vi "SERIAL_BufferLoop.vi"(11 "navX DevRef":T1={"SerialPortRef"={"DevStatus"={"status"=FALSE, "code"=0, "source"=""}, "Serial Port Name"=""}, "Board Information"={"WhoAmI (50 | 0x32)"=0, "Board Revision"=0, "Firmware Major Version"=0, "Firmware Minor Version"=0}, "Status"={"Update Rate Hz"=0, "Accelerometer Full-Scale Range"=0, "Gyro Full-Scale Range"=0, "NAVX_OP_STATUS"=0, "NAVX_CAL_STATUS"=0, "NAVX_SELFTEST_STATUS"=0, "NAVX_SENSOR_STATUS"={"MOVING"=FALSE, "YAW_STABLE"=FALSE, "MAG_DISTURBANCE"=FALSE, "ALTITUDE_VALID"=FALSE, "SEALEVEL_PRESS_SET"=FALSE, "FUSED_HEADING_VALID"=FALSE}}, "Offsets"={"Yaw"=0.0, "Quat W"=0.0, "Quat X"=0.0, "Quat Y"=0.0, "Quat Z"=0.0}, "Update Rate (4Hz-60Hz)"=50, "Nav6Mode (YPR)"=enum."YPR", "refnum name"="", "error"={"status"=FALSE, "code"=0, "source"=""}, "Loop VI Refnum"=refnum} {"Status"."NAVX_OP_STATUS" items=["INITIALIZING", "SELFTEST_IN_PROGRESS", "ERROR", "IMU_AUTOCAL_IN_PROGRESS", "NORMAL"]; "Status"."NAVX_CAL_STATUS" items=["IMU_CAL_STATE_MASK"=3, "IMU_CAL_INPROGRESS"=0, "IMU_CAL_ACCUMULATE"=1, "IMU_CAL_COMPLETE"=2, "MAG_CAL_COMPLETE"=4, "BARO_CAL_COMPLETE"=8]}) -> ()   [LabVIEW 2014, in "navX-MXP IMU.lvlib"]
uses:
  navX-MXP IMU.lvlib
  Internal/navX Serial DevRef.ctl
  <vilib>/Rock Robotics/WPI/SerialPort/WPI_SerialPortRef.ctl
  COMMON/TypeDefs/Data TypeDefs/navX Board Information.ctl
  COMMON/TypeDefs/Data TypeDefs/navX Status Data.ctl
  COMMON/TypeDefs/Value TypeDefs/navX NAVX_OP_STATUS.ctl
  COMMON/TypeDefs/Value TypeDefs/navX NAVX_CAL_STATUS.ctl
  COMMON/TypeDefs/Value TypeDefs/navX NAVX_SENSOR_STATUS.ctl
  TypeDefs/navX Serial Mode.ctl
  <vilib>/Platform/TimedLoop/XDataNode/timing_clust.ctl
  <vilib>/Platform/TimedLoop/XDataNode/nitl_modes.ctl
  <vilib>/Platform/TimedLoop/XDataNode/wakeup.ctl
  <vilib>/platform/TimedLoop/XDataNode/XDataNode.xnode
  <vilib>/Platform/TimedLoop/XDataNode/XDNodeRunTimeDep.lvlib
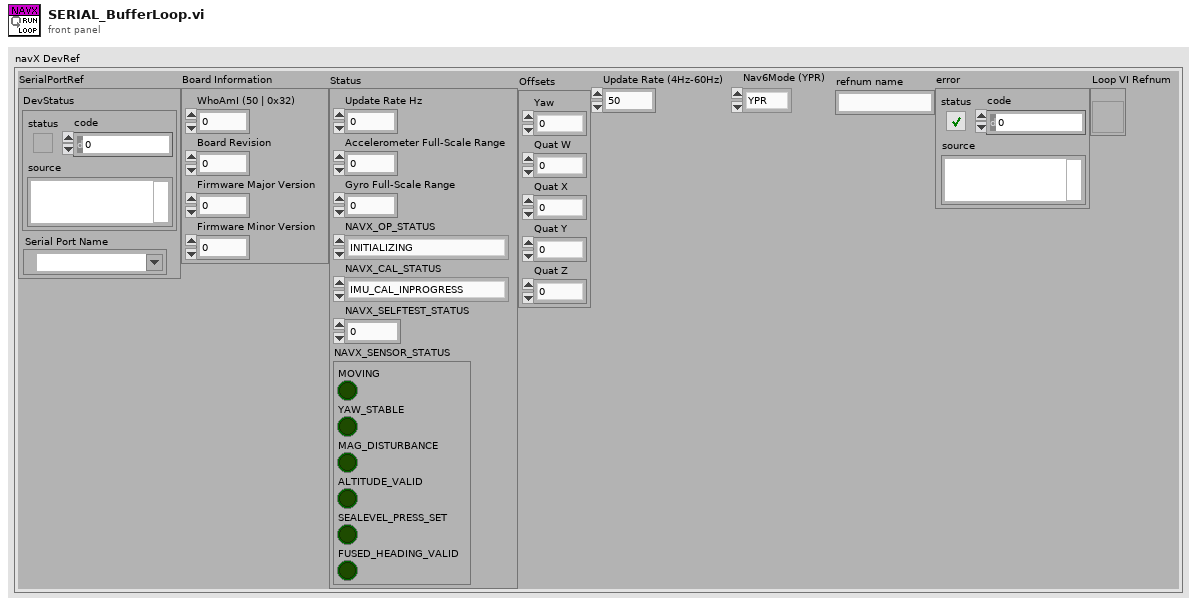
[diagram p1: front panel]
types:
  T1 = typedef "navX-MXP IMU.lvlib/navX Serial DevRef.ctl" = cluster{"SerialPortRef":T2, "Board Information":T3, "Status":T4, "Offsets":cluster{"Yaw":dbl, "Quat W":dbl, "Quat X":dbl, "Quat Y":dbl, "Quat Z":dbl}, "Update Rate (4Hz-60Hz)":u8, "Nav6Mode (YPR)":T8, "refnum name":string, "error":errorcluster, "Loop VI Refnum":refnum<vi>}
  T2 = typedef "WPI_SerialPortRef.ctl" = cluster{"DevStatus":errorcluster, "Serial Port Name":refnum<visa-resource-name>}
  T3 = typedef "navX-MXP IMU.lvlib/navX Board Information.ctl" = cluster{"WhoAmI (50 | 0x32)":u8, "Board Revision":u8, "Firmware Major Version":u8, "Firmware Minor Version":u8}
  T4 = typedef "navX-MXP IMU.lvlib/navX Status Data.ctl" = cluster{"Update Rate Hz":u8, "Accelerometer Full-Scale Range":u8, "Gyro Full-Scale Range":u16, "NAVX_OP_STATUS":T5, "NAVX_CAL_STATUS":T6, "NAVX_SELFTEST_STATUS":u8, "NAVX_SENSOR_STATUS":T7}
  T5 = typedef "navX-MXP IMU.lvlib/navX NAVX_OP_STATUS.ctl" = u8
  T6 = typedef "navX-MXP IMU.lvlib/navX NAVX_CAL_STATUS.ctl" = u8
  T7 = typedef "navX-MXP IMU.lvlib/navX NAVX_SENSOR_STATUS.ctl" = cluster{"MOVING":bool, "YAW_STABLE":bool, "MAG_DISTURBANCE":bool, "ALTITUDE_VALID":bool, "SEALEVEL_PRESS_SET":bool, "FUSED_HEADING_VALID":bool}
  T8 = typedef "navX-MXP IMU.lvlib/navX Serial Mode.ctl" = enum16{"YPR", "Gyro", "Quaternion"}
  T9 = typedef "XDNodeRunTimeDep.lvlib/timing_clust.ctl" = cluster{"Expected End [f-1]":u64, "Actual End [f-1]":u64, "Finished Late? [f-1]":bool, "Expected End [i-1]":u64, "Actual End [i-1]":u64, "Finished Late? [i-1]":bool, "Expected Start [i]":u64, "Actual Start [i]":u64, "Expected Start [f]":u64, "Actual Start [f]":u64, "Source Name":string, "Structure Name":string, "Period":i64, "Deadline":i64, "Offset":i64, "Start":i64, "Priority":i32, "Timeout":i32, "Mode":T10, "Wakeup Reason":T11, "Error":errorcluster, "Source Type":string, "Secondary Source Type":string, "Global End Time":u64, "Global Start Time":u64, "Frame Duration":u64, "Iteration Duration":u64, "Assigned CPU":i32, "I/O Scan Engine Mode":u32}
  T10 = typedef "XDNodeRunTimeDep.lvlib/nitl_modes.ctl" = enum32{"No Change", "Process missed periods, maintain original phase", "Discard missed periods, maintain original phase", "Process missed periods, ignore original phase", "Discard missed periods, ignore original phase"}
  T11 = typedef "XDNodeRunTimeDep.lvlib/wakeup.ctl" = enum32{"Normal", "Aborted", "Asynchronous wakeup", "Timing source error", "Timed loop error", "Timeout"}
  T12 = typedef "navX-MXP IMU.lvlib/navX YPRH Data.ctl" = cluster{"Yaw":dbl, "Pitch":dbl, "Roll":dbl, "Heading":dbl}
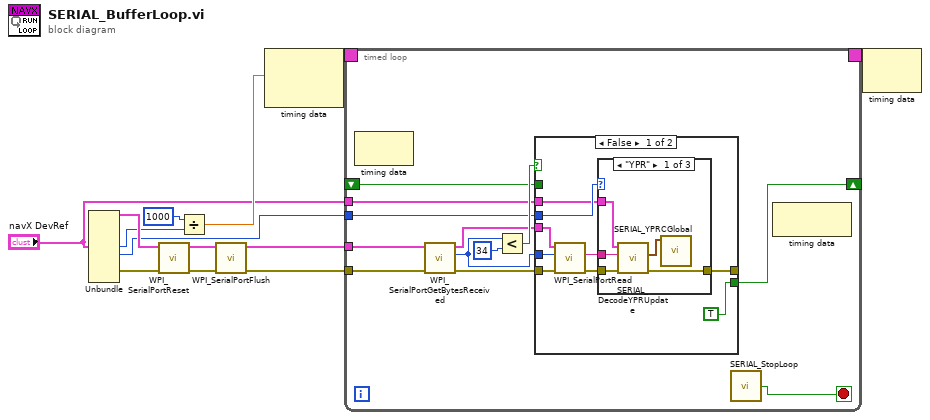
[diagram p0: block diagram]
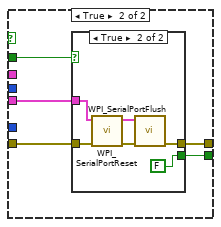
[diagram p4: hidden frame]
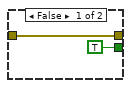
[diagram p5: hidden frame]
diagram:
  n1 = Unbundle("navX DevRef") -> ("SerialPortRef"=w13:T2, "Update Rate (4Hz-60Hz)"=w3:u8, "Nav6Mode (YPR)"=w5:T8, "error"=w4:errorcluster)  [unwired: 5 out]
  n2 = call <vilib>:"WPI_SerialPortReset.vi"("error in (no error)"=w4, "SerialPortRef"=w13) -> ("error out"=w12:errorcluster, "SerialPortRef"=w11:T2)  [unwired: 8 in]
  n3 = Divide(x=1000, y=w3) -> (x/y=w7:dbl)
  n4 = call <vilib>:"WPI_SerialPortFlush.vi"("error in (no error)"=w12, "SerialPortRef"=w11) -> ("error out"=w1:errorcluster, "SerialPortRef"=w6:T2)  [unwired: 8 in]
  n5 = node-c288(w7) -> (w10:T9)  [unwired: 1 in]
  n6 = timed-loop {
    timing: w10 -> [_]
    timing-out: [_] -> w9
    tunnel: w6 -> [w25]
    shift-right: [w19] -> _
    shift-left: _ -> [w22]
    tunnel: w5 -> [w17]
    tunnel: "navX DevRef" -> [w16]
    tunnel: w1 -> [w14]
    stop <- w15 stop-if-true
    n7 = node-c288() -> ()  [unwired: 1 in, 1 out]
    n8 = call <vilib>:"WPI_SerialPortGetBytesReceived.vi"("error in (no error)"=w14, "SerialPortRef"=w25) -> ("error out"=w20:errorcluster, "Bytes at Port"=w18:u32, "SerialPortRef"=w21:T2)  [unwired: 7 in]
    n9 = Less?(x=w18, y=u32 34) -> (x < y?=w23:bool)
    n10 = case shown="False" w23 {
      tunnel: w22 -> [_ w46]
      tunnel: w21 -> [w33 w45]
      tunnel: w20 -> [w32 w44]
      tunnel: [TRUE w43] -> w19
      tunnel: w18 -> [w31 _]
      tunnel: w17 -> [w28 _]
      tunnel: [w27 w42] -> _
      tunnel: w16 -> [w26 _]
      frame False {
        n11 = call <vilib>:"WPI_SerialPortRead.vi"("error in (no error)"=w32, "Num Bytes to Read"=w31, "SerialPortRef"=w33) -> ("error out"=w29:errorcluster, "Buffer"=w30:string)  [unwired: 6 in, 1 out]
        n12 = case shown="\"YPR\"" w28 {
          tunnel: w30 -> [w36 _ _]
          tunnel: w29 -> [w39 w40 w41]
          tunnel: [w38 w40 w41] -> w27
          tunnel: w26 -> [w35 _ _]
          frame "YPR" {
            n13 = call "SERIAL_DecodeYPRUpdate.vi"("error in"=w39, "Buffer"=w36, "navX DevRef"=w35) -> ("error out"=w38:errorcluster, "YPR Update"=w37:T12)  [unwired: 5 in, 2 out]
            n14 = call "SERIAL_YPRCGlobal.vi"("YPRH"=w37) -> ()  [unwired: 9 in, 2 out]
          }
          frame "Gyro" {
          }
          frame "Quaternion" {
          }
        }
      }
      frame True {
        n15 = case shown="True" w46 {
          tunnel: w45 -> [_ w52]
          tunnel: w44 -> [w47 w51]
          tunnel: [TRUE FALSE] -> w43
          tunnel: [w47 w49] -> w42
          frame False {
          }
          frame True {
            n16 = call <vilib>:"WPI_SerialPortReset.vi"("error in (no error)"=w51, "SerialPortRef"=w52) -> ("error out"=w54:errorcluster, "SerialPortRef"=w53:T2)  [unwired: 8 in]
            n17 = call <vilib>:"WPI_SerialPortFlush.vi"("error in (no error)"=w54, "SerialPortRef"=w53) -> ("error out"=w49:errorcluster)  [unwired: 8 in, 1 out]
          }
        }
      }
    }
    n18 = call "SERIAL_StopLoop.vi"() -> ("Stop?"=w15:bool)  [unwired: 2 in]
    n19 = node-c288() -> ()  [unwired: 1 in, 1 out]
  }
  n20 = node-c288(w9) -> ()  [unwired: 1 out]
